vi "Calculate Frame Per Second.vi"(7 "Execeeded 1sec":bool, 8 "Previous Buffer Number":u32, 9 "Run start time":timestamp, 10 "Display Frames per Second in":u32, 11 "Current Buffer Number":u32) -> (0 "Updated Buffer":u32, 1 "Updated Start Time":timestamp, 2 "Display Frames per Second out":u32)   [LabVIEW 2021, in "ImageRendering.lvlib"]
uses:
  ImageRendering.lvlib
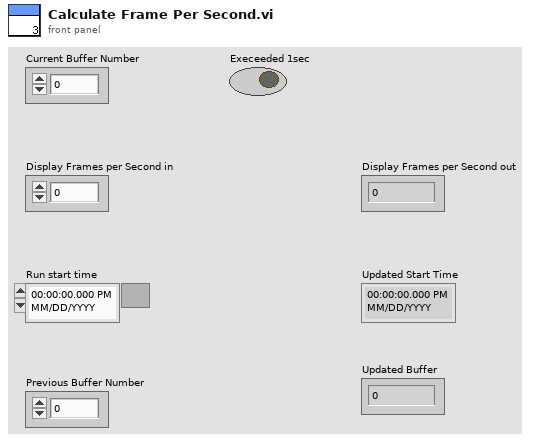
[diagram p1: front panel]
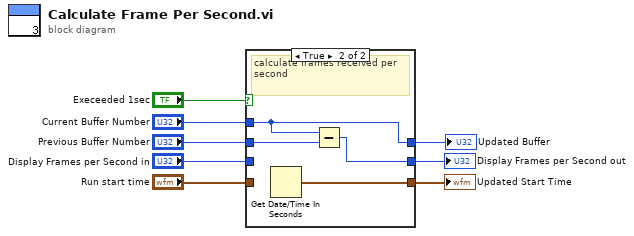
[diagram p0: block diagram]
diagram:
  n1 = case shown="True" "Execeeded 1sec" {
    tunnel: "Previous Buffer Number" -> [w9 w15]
    tunnel: [w11 w14] -> w5
    tunnel: "Run start time" -> [w11 _]
    tunnel: [w10 w13] -> w6
    tunnel: "Display Frames per Second in" -> [w10 _]
    tunnel: "Current Buffer Number" -> [_ w12]
    tunnel: [w9 w12] -> w1
    frame False {
    }
    frame True {
      # "calculate frames received per second"
      n2 = Get Date/Time In Seconds() -> (seconds since 1Jan1904=w14:timestamp)
      n3 = Subtract(x=w12, y=w15) -> (x-y=w13:u32)
    }
  }
  "Display Frames per Second out" <- w6
  "Updated Start Time" <- w5
  "Updated Buffer" <- w1
